vi "hardwareInfo.vi"() -> (0 "error out":errorcluster, 3 "response":string)   [LabVIEW 2017]
uses:
  <vilib>/httpClient/LabVIEWHTTPClient.lvlib
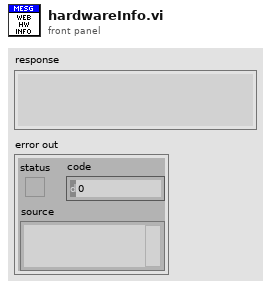
[diagram p1: front panel]
types:
  T1 = typedef "LabVIEWHTTPClient.lvlib/ClientHandle.ctl" = refnum<k1>
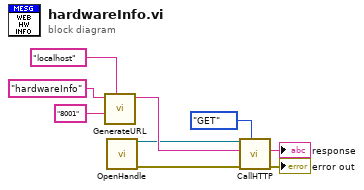
[diagram p0: block diagram]
diagram:
  n1 = call "GenerateURL.vi"("host"="localhost", "port"="8001", "method"="hardwareInfo") -> ("url"=w8:string)  [unwired: 7 in, 1 out]
  n2 = call <vilib>:"OpenHandle.vi"() -> ("client handle out"=w7:T1, "error out"=w6:errorcluster)  [unwired: 14 in]
  n3 = call "CallHTTP.vi"("Enum"=enum16{"GET", "POST", "DELETE"}."GET", "error in (no error)"=w6, "url"=w8, "client handle"=w7) -> ("error out"=→"error out":errorcluster, "response"=→"response":string)  [unwired: 4 in, 2 out]
